vi "Update Water Level.vi"(8 "error in (no error)":errorcluster, 10 "Water Level":dbl, 11 "Evaporative Cooler":refnum<class "Evaporative Cooler.lvclass">) -> (0 "error out":errorcluster, 3 "Evaporative Cooler":refnum<class "Evaporative Cooler.lvclass">)   [LabVIEW 2025, in "Evaporative Cooler.lvlib" / "Evaporative Cooler.lvclass"]
doc: "This method sends a message to the controller letting it know information about the water level in the basin."
uses:
  Evaporative Cooler/Evaporative Cooler/Evaporative Cooler.lvclass
  C:/Program Files/National Instruments/LabVIEW 2025/ProjectTemplates/Source/Core/Feedback Evaporative Cooler/Cooler/Cooler/Cooler.lvclass
  <vilib>/ActorFramework/Message Enqueuer/Message Enqueuer.lvclass
  Cooler.lvclass/Cooler.ctl
  Evaporative Cooler Controller/Update Water Level Msg/Update Water Level Msg.lvclass/Update Water Level Msg.ctl
  <vilib>/ActorFramework/Message Enqueuer/Message Enqueuer.lvclass/Message Enqueuer.ctl
  <vilib>/ActorFramework/Message Enqueuer/Enqueue.vi
  Evaporative Cooler Controller/Update Water Level Msg/Update Water Level Msg.lvclass
  C:/Program Files/National Instruments/LabVIEW 2025/vi.lib/ActorFramework/Message/Message.lvclass
  <vilib>/ActorFramework/Message Priority Queue/Priority Enqueue.vi
  Cooler.lvclass
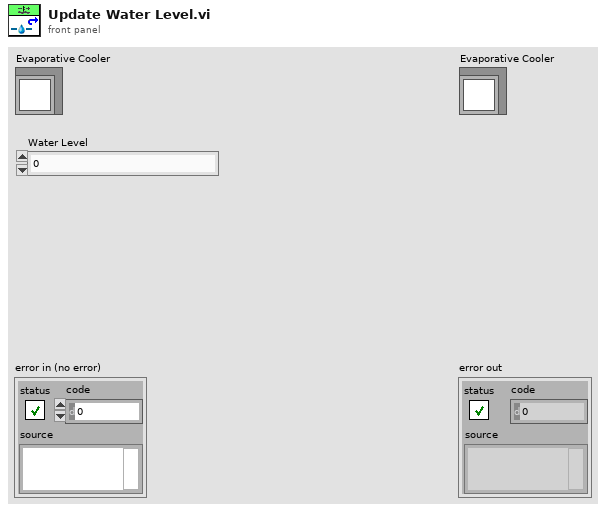
[diagram p1: front panel]
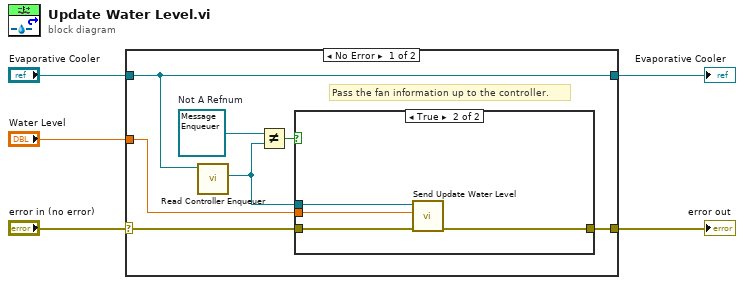
[diagram p0: block diagram]
diagram:
  n1 = case shown="No Error" "error in (no error)" {
    selector: "error in (no error)" -> [w11 w19]
    tunnel: [w10 w19] -> w4
    tunnel: [w12 w18] -> w2
    tunnel: "Evaporative Cooler" -> [w12 w18]
    tunnel: "Water Level" -> [w6 _]
    frame No Error {
      w8 = refnum<class "Message Enqueuer.lvclass"> refnum  # Not A Refnum
      # "Pass the fan information up to the controller."
      n2 = call "Read Controller Enqueuer.vi"("Cooler"=w12) -> ("Controller Enqueuer"=w9:refnum<class "Message Enqueuer.lvclass">)  [unwired: 10 in]
      n3 = Not Equal?(x=w8, y=w9) -> (x != y?=w7:bool)
      n4 = case shown="True" w7 {
        tunnel: w9 -> [_ w17]
        tunnel: w11 -> [w13 w16]
        tunnel: [w13 w15] -> w10
        tunnel: w6 -> [_ w14]
        frame False {
        }
        frame True {
          n5 = call "Send Update Water Level.vi"("error in (no error)"=w16, "Water Level"=w14, "Message Enqueuer"=w17) -> ("error out"=w15:errorcluster)  [unwired: 8 in]
        }
      }
    }
    frame Error {
    }
  }
  "error out" <- w4
  "Evaporative Cooler" <- w2
